vi "nirviDutyCycleLatch.vi"(0 "current_accum_state":fxp<+,32,0>, 1 "reset":bool, 5 "phase offset":fxp<+,32,0>, 7 "duty cycle":fxp<+,32,0>) -> (6 "hi/lo?":bool)   [LabVIEW 2017]
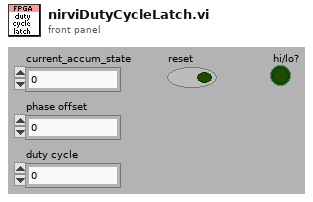
[diagram p1: front panel]
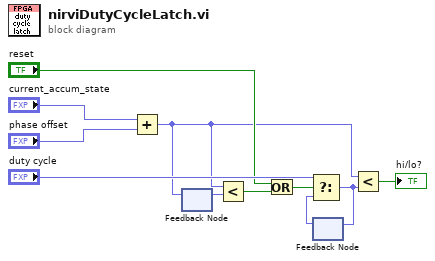
[diagram p0: block diagram]
diagram:
  n1 = Add(x="current_accum_state", y="phase offset") -> (x+y=w1:fxp<+,32,0>)
  n2 = feedback-in #1(w1) -> ()
  n3 = feedback #1() -> (w5:fxp<+,32,0>)  [unwired: 1 out]
  n4 = Less?(x=w1, y=w5) -> (x < y?=w2:bool)
  n5 = Or(x="reset", y=w2) -> (x .or. y?=w8:bool)
  n6 = feedback #2() -> (w6:fxp<+,32,0>)  [unwired: 1 out]
  n7 = Select(t="duty cycle", s=w8, f=w6) -> (s? t:f=w7:fxp<+,32,0>)
  n8 = feedback-in #2(w7) -> ()
  n9 = Less?(x=w1, y=w7) -> (x < y?=→"hi/lo?":bool)
